vi "recon_zern_ramIO_MATLAB.vi"(0 "Number of Phase":u32=2, 1 "Number for average":u32=2, 2 "Crop Size of image":u32=384, 3 "Background Value":u32=290, 4 "Zernike Order":u32=15, 5 "error in (no error)":errorcluster, 6 "Use GPU":bool=TRUE, 7 "Iteration Number":u32=10, 9 "Gamma Value":dbl=1e-06, 11 "Show Input":bool, 12 "Path Out":path=path "D:/Data", 13 "Show Recon":bool=TRUE) -> (14 "Zern coef out":sgl[](array[numeric]), 16 "Time cost (s)":dbl, 17 "RMSE Value":dbl, 19 "error out":errorcluster)   [LabVIEW 2018]
panel:
  in  "imgNumN":u32=10
  in  "imgSizeY":u32=512
  in  "imgSizeX":u32=512
  in  "imgsIn":sgl[][](array[numeric])
  in  "coeffsIn":sgl[][](array[numeric])
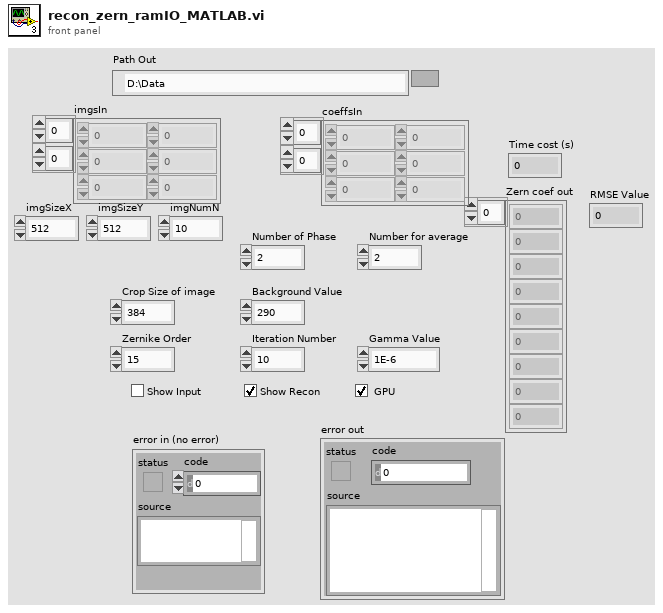
[diagram p1: front panel]
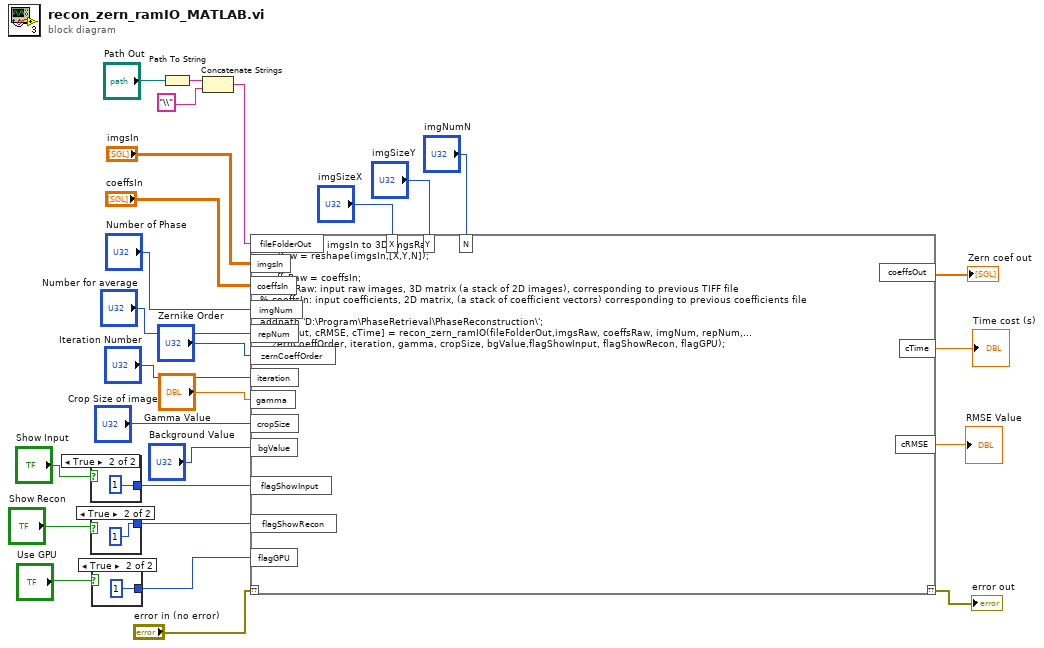
[diagram p0: block diagram]
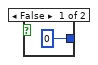
[diagram p2: hidden frame]
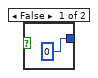
[diagram p3: hidden frame]
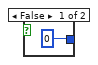
[diagram p4: hidden frame]
diagram:
  n1 = case shown="True" "Show Input" {
    tunnel: [0 1] -> w20
    frame False {
    }
    frame True {
    }
  }
  n2 = case shown="True" "Show Recon" {
    tunnel: [0 1] -> w19
    frame False {
    }
    frame True {
    }
  }
  n3 = case shown="True" "Use GPU" {
    tunnel: [0 1] -> w18
    frame False {
    }
    frame True {
    }
  }
  n4 = Path To String(path="Path Out") -> (string=w10:string)
  n5 = Concatenate Strings(w10, "\\") -> (w9:string)
  n6 = script code="% convert 2D imgsIn to 3D imgsRaw\nimgRaw = reshape(imgsIn,[X,Y,N]);\n\ncoeffsRaw = coeffsIn;\n% imgsRaw: input raw images, 3D matrix (a stack of 2D images), corresponding to previous TIFF file\n% coeffsIn: input coefficients, 2D matrix, (a stack of coefficient vectors) corresponding to previous coefficients file\nclose all;\naddpath 'D:\\Program\\PhaseRetrieval\\PhaseReconstruction\\';\n[coeffsOut, cRMSE, cTime] = recon_zern_ramIO(fileFolderOut,imgsRaw, coeffsRaw, imgNum, repNum,...\n    zernCoeffOrder, iteration, gamma, cropSize, bgValue,flagShowInput, flagShowRecon, flagGPU);"("??"="error in (no error)", "fileFolderOut"=w9, "imgNum"="Number of Phase", "repNum"="Number for average", "zernCoeffOrder"="Zernike Order", "iteration"="Iteration Number", "gamma"="Gamma Value", "cropSize"="Crop Size of image", "bgValue"="Background Value", "flagShowInput"=w20, "flagShowRecon"=w19, "flagGPU"=w18, "imgsIn"="imgsIn", "coeffsIn"="coeffsIn", "X"="imgSizeX", "Y"="imgSizeY", "N"="imgNumN") -> ("??"=→"error out":errorcluster, "coeffsOut"=→"Zern coef out":dbl[], "cTime"=→"Time cost (s)":dbl, "cRMSE"=→"RMSE Value":dbl)
